vi "ALTS-2015 Serial Task Enqueue Handler FGV.vi"(7 "Command":T2=enum."Get Status", 8 "Error In":errorcluster, 11 "Task Details In":T3) -> (0 "Error Out":errorcluster, 1 "Task Details Out":T3, 3 "Operation":T1=enum."No Operation")   [LabVIEW 2013]
uses:
  Controls/ALTS-2015 Serial Details.ctl
  Controls/ALTS-2015 Robot Tasks.ctl
  Controls/ALTS-2015 Station Cluster.ctl
  Controls/ALTS-2015 Serial DB Details.ctl
  Controls/ALTS-2015 Serial Task Handler FGV-Command.ctl
  Controls/ALTS-2015 Serial Task Handler FGV-Operation.ctl
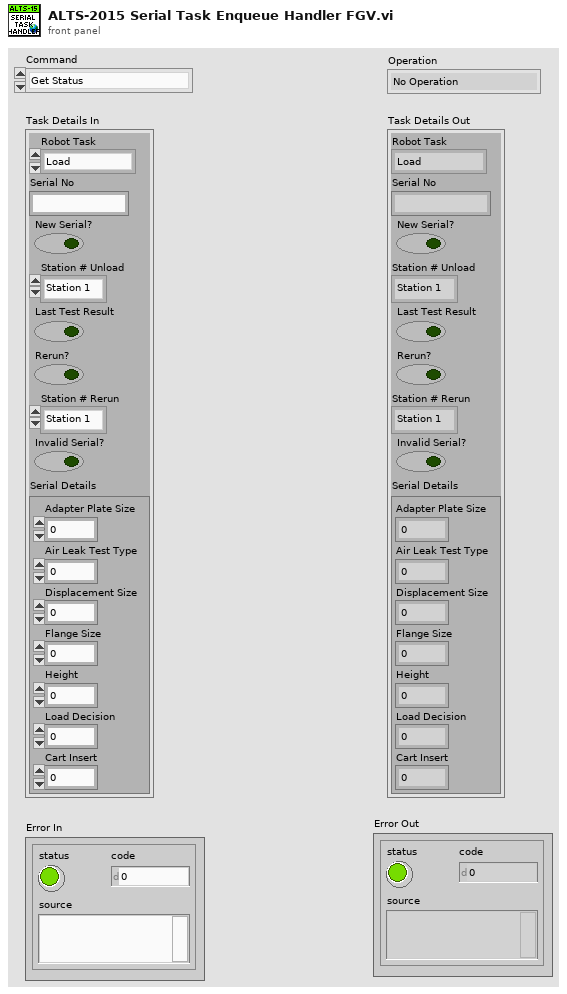
[diagram p1: front panel]
types:
  T1 = typedef "ALTS-2015 Serial Task Handler FGV-Operation.ctl" = enum16{"Replace/Insert", "No Operation"}
  T2 = typedef "ALTS-2015 Serial Task Handler FGV-Command.ctl" = enum16{"Set Replace/Insert Falg", "Get Status", "Reset Flag"}
  T3 = typedef "ALTS-2015 Serial Details.ctl" = cluster{"Robot Task":T4, "Serial No":string, "New Serial?":bool, "Station # Unload":T5, "Last Test Result":bool, "Rerun?":bool, "Station # Rerun":T5, "Invalid Serial?":bool, "Serial Details":T6}
  T4 = typedef "ALTS-2015 Robot Tasks.ctl" = enum16{"Load", "Unload", "Rerun", "Invalid Serial"}
  T5 = typedef "ALTS-2015 Station Cluster.ctl" = enum16{"Station 1", "Station 2", "Station 3", "Station 4"}
  T6 = typedef "ALTS-2015 Serial DB Details.ctl" = cluster{"Adapter Plate Size":i32, "Air Leak Test Type ":i32, "Displacement Size":i32, "Flange Size":i32, "Height":i32, "Load Decision":i32, "Cart Insert":i32}
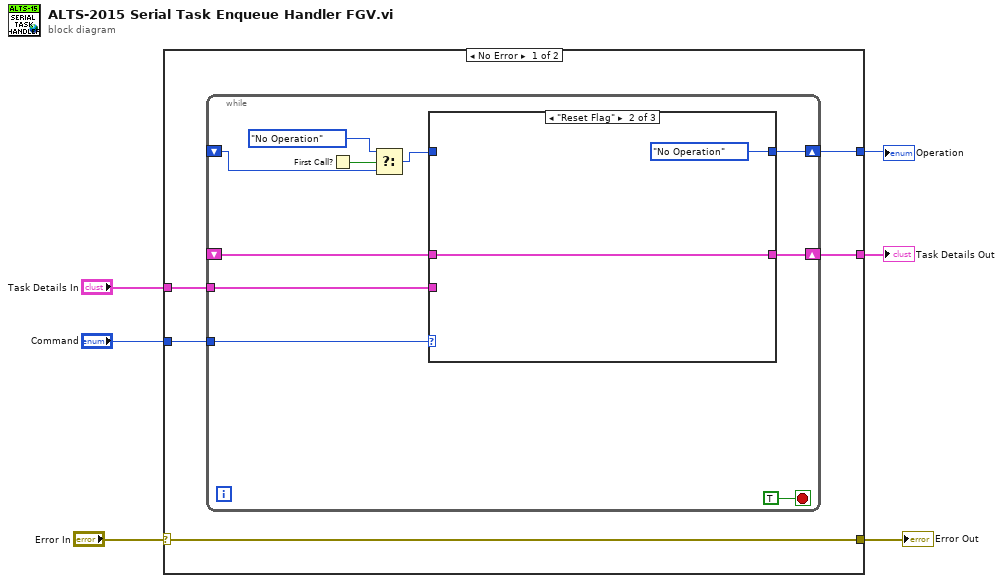
[diagram p0: block diagram]
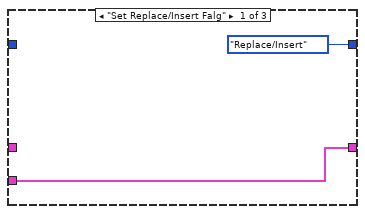
[diagram p2: hidden frame]
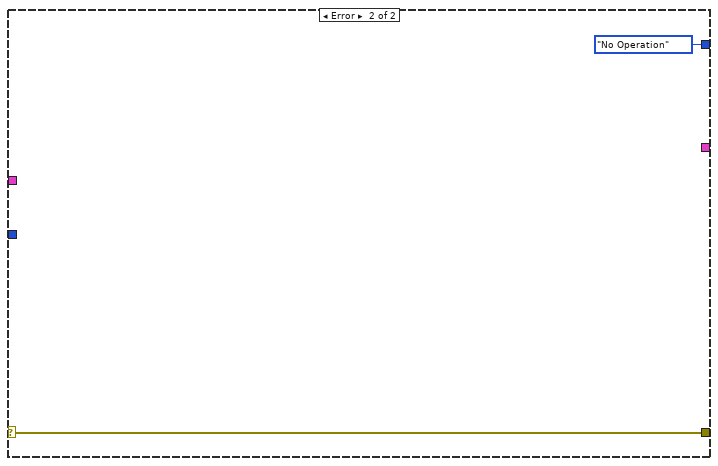
[diagram p4: hidden frame]
diagram:
  n1 = case shown="No Error" "Error In" {
    selector: "Error In" -> [w7 w29]
    tunnel: "Command" -> [w11 _]
    tunnel: "Task Details In" -> [w10 _]
    tunnel: [w9 _] -> w4
    tunnel: [w8 ALTS-2015_Serial_Task_Handler_FGV-Operation."No Operation"] -> w3
    tunnel: [w7 w29] -> w1
    frame No Error {
      n2 = while {
        tunnel: w11 -> [w20]
        shift-right: [w14] -> w8
        shift-left: _ -> [w13]
        tunnel: w10 -> [w17]
        shift-right: [w18] -> w9
        shift-left: _ -> [w16]
        stop <- TRUE stop-if-true
        n3 = First Call?() -> (First Call?: T/F=w19:bool)
        n4 = Select(t=ALTS-2015_Serial_Task_Handler_FGV-Operation."No Operation", s=w19, f=w13) -> (s? t:f=w15:T1)
        n5 = case shown="\"Reset Flag\"" w20 {
          tunnel: w15 -> [_ _ w26]
          tunnel: [ALTS-2015_Serial_Task_Handler_FGV-Operation."Replace/Insert" ALTS-2015_Serial_Task_Handler_FGV-Operation."No Operation" w26] -> w14
          tunnel: [w23 w25 w27] -> w18
          tunnel: w17 -> [w23 _ _]
          tunnel: w16 -> [_ w25 w27]
          frame "Set Replace/Insert Falg" {
          }
          frame "Reset Flag" {
          }
          frame "Get Status" {
          }
        }
      }
    }
    frame Error {
    }
  }
  "Task Details Out" <- w4
  "Error Out" <- w1
  "Operation" <- w3
